vi "csuOpen.vi"() -> (4 "VISA OUT":refnum<visa-resource-name>, 15 "error out":errorcluster)   [LabVIEW 2017]
doc: "VI initializes and configues the MAC5000; the user chooses whether communication with the MAC5000 occurs over the Serial Port(RS232) or the USB port. This VI should be run once at the beginning of a larger program.\n\nNote: \nSerial Port communication occurs over Serial Port 1; if the user wants to use a different Serial Port the VISA Resource name needs to be changed in the block diagram from ASRL1::INSTR to ASRL#::INSTR where # is the number of the Serial Port.\nTo use USB communication, the user needs to set up the VISA protocol using the VISA driver development wizard. After setting up the VISA driver, the user needs to enter the correct VISA resource name in the block diagram. Note the VISA resource name is specific to a particular USB Bus; if the MAC5000 is plugged into another USB bus the user needs to set up the VISA resource name again."
uses:
  <vilib>/Platform/TimedLoop/XDataNode/timing_clust.ctl
  <vilib>/Platform/TimedLoop/XDataNode/nitl_modes.ctl
  <vilib>/Platform/TimedLoop/XDataNode/wakeup.ctl
  globalDevices.vi
  <vilib>/Instr/_visa.llb/VISA Configure Serial Port (Instr).vi
  <vilib>/platform/TimedLoop/XDataNode/XDataNode.xnode
  <vilib>/Platform/TimedLoop/XDataNode/XDNodeRunTimeDep.lvlib
panel:
  out "Raw Response":string
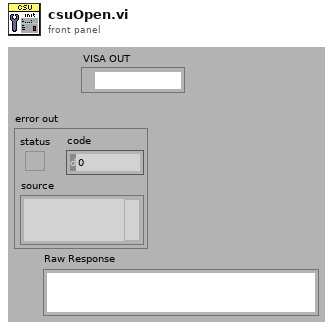
[diagram p1: front panel]
types:
  T1 = typedef "XDNodeRunTimeDep.lvlib/timing_clust.ctl" = cluster{"Expected End [f-1]":u64, "Actual End [f-1]":u64, "Finished Late? [f-1]":bool, "Expected End [i-1]":u64, "Actual End [i-1]":u64, "Finished Late? [i-1]":bool, "Expected Start [i]":u64, "Actual Start [i]":u64, "Expected Start [f]":u64, "Actual Start [f]":u64, "Source Name":string, "Structure Name":string, "Period":i64, "Deadline":i64, "Offset":i64, "Start":i64, "Priority":i32, "Timeout":i32, "Mode":T2, "Wakeup Reason":T3, "Error":errorcluster, "Source Type":string, "Secondary Source Type":string, "Global End Time":u64, "Global Start Time":u64, "Frame Duration":u64, "Iteration Duration":u64, "Assigned CPU":i32, "I/O Scan Engine Mode":u32}
  T2 = typedef "XDNodeRunTimeDep.lvlib/nitl_modes.ctl" = enum32{"No Change", "Process missed periods, maintain original phase", "Discard missed periods, maintain original phase", "Process missed periods, ignore original phase", "Discard missed periods, ignore original phase"}
  T3 = typedef "XDNodeRunTimeDep.lvlib/wakeup.ctl" = enum32{"Normal", "Aborted", "Asynchronous wakeup", "Timing source error", "Timed loop error", "Timeout"}
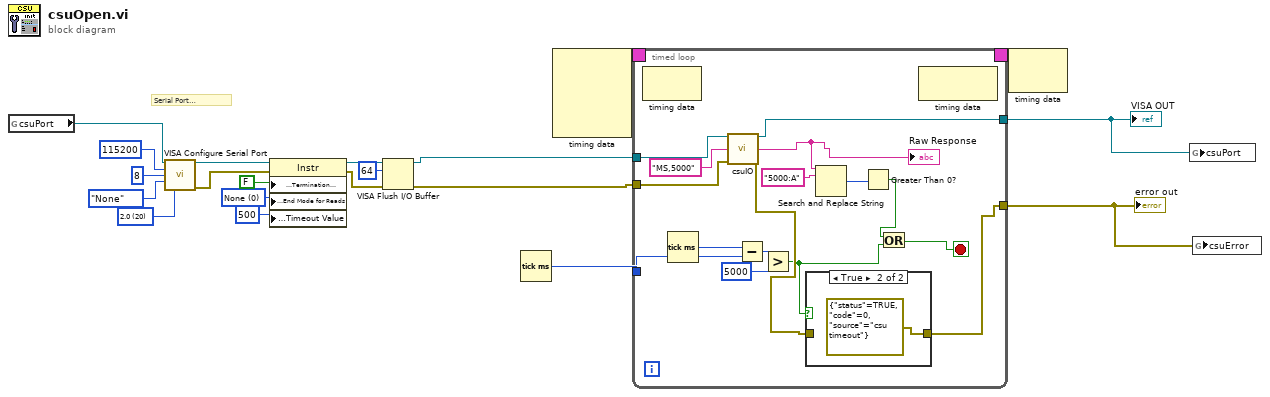
[diagram p0: block diagram]
diagram:
  w9 = u16 20 items=["1.0"=10, "1.5"=15, "2.0"=20] ("stop bits (10: 1 bit)")
  w16 = u16 0 items=["None", "LastBit", "TermChar"] ("Serial Settings:Serial End Mode for Reads")
  # "Serial Port Configuration"
  n1 = global read "globalDevices.vi" "csuPort"() -> (w3:refnum<visa-resource-name>)
  n2 = call-poly "VISA Configure Serial Port"("VISA resource name"=w3, "baud rate (9600)"=u32 115200, "data bits (8)"=u16 8, "parity (0:none)"=enum16{"None", "Odd", "Even", "Mark", "Space"}."None", "stop bits (10: 1 bit)"=w9) -> ("VISA resource name out"=w14:refnum<visa-resource-name>, "error out"=w13:errorcluster)  [unwired: 9 in]
  n3 = property class="Instr"(reference=w14, error in=w13, "Message Based Settings:Termination Character Enable"=FALSE, "Serial Settings:End Mode for Reads"=w16, "General Settings:Timeout Value"=u32 500) -> (reference out=w11:refnum<visa-resource-name>, error out=w10:errorcluster)
  n4 = VISA Flush I/O Buffer(VISA resource name=w11, mask (16)=u16 64, error in (no error)=w10) -> (VISA resource name out=w8:refnum<visa-resource-name>, error out=w5:errorcluster)
  n5 = Tick Count (ms)() -> (millisecond timer value=w4:u32)
  n6 = node-c288() -> (w7:T1)  [unwired: 4 in]
  n7 = timed-loop {
    timing: w7 -> [_]
    timing-out: [_] -> w6
    tunnel: w8 -> [w36]
    tunnel: w5 -> [w31]
    tunnel: [w25] -> w1
    tunnel: w4 -> [w30]
    tunnel: [w21] -> w2
    stop <- w24 stop-if-true
    n8 = node-c288() -> ()  [unwired: 1 in, 1 out]
    n9 = Tick Count (ms)() -> (millisecond timer value=w29:u32)
    n10 = call "csuIO.vi"("VISA  IN"=w36, "Command (to ctlr)"="MS,5000", "error in"=w31) -> ("VISA OUT"=w21:refnum<visa-resource-name>, "Raw Response"=w34:string, "error out"=w26:errorcluster)  [unwired: 9 in, 1 out]
    "Raw Response" <- w34
    n11 = Subtract(x=w29, y=w30) -> (x-y=w28:u32)
    n12 = Greater?(x=w28, y=u32 5000) -> (0:w22:bool)
    n13 = case shown="True" w22 {
      tunnel: w26 -> [w37 _]
      tunnel: [w37 errorcluster {"status"=TRUE, "code"=0, "source"="csu timeout"} ("error constant")] -> w25
      frame False {
      }
      frame True {
      }
    }
    n14 = Search and Replace String(input string=w34, search string="5000:A" ("y")) -> (number of replacements=w32:i32)  [unwired: 6 in, 3 out]
    n15 = Greater Than 0?(x=w32) -> (x > 0?=w23:bool)
    n16 = Or(x=w23, y=w22) -> (x .or. y?=w24:bool)
    n17 = node-c288() -> ()  [unwired: 1 in, 1 out]
  }
  "error out" <- w1
  "VISA OUT" <- w2
  n18 = node-c288(w6) -> ()  [unwired: 1 out]
  n19 = global write "globalDevices.vi" "csuPort"(w2) -> ()
  n20 = global write "globalDevices.vi" "csuError"(w1) -> ()
